vi "Get Installed Sections.vi"(8 "error in (no error)":errorcluster, 9 "Cached (F)":bool, 11 "Session in":refnum<k21>) -> (0 "error out":errorcluster, 2 "Software Components":T1[](array[typedef]) {"Visibility Type" items=["standard", "hidden", "system", "unknown", "startup", "image"]}, 3 "Session out":refnum<k21>)   [LabVIEW 2014, in "nisyscfg.lvlib"]
uses:
  nisyscfg.lvlib
  Software Extended.ctl
  Component Type.ctl
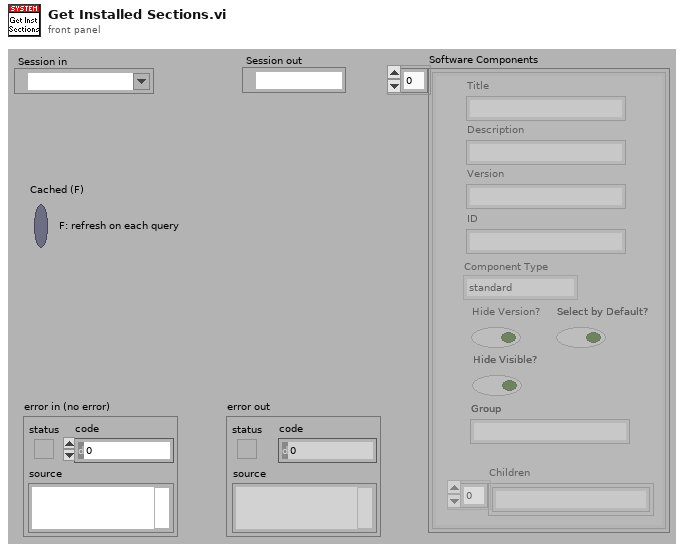
[diagram p1: front panel]
types:
  T1 = typedef "nisyscfg.lvlib/Software Extended.ctl" = cluster{"Description":string, "ID":string, "Version":string, "Title":string, "Visibility Type":T2, "Hide Version?":bool, "Children":string[], "Select by Default?":bool, "Hide Visible?":bool, "Group":string}
  T2 = typedef "nisyscfg.lvlib/Component Type.ctl" = u32
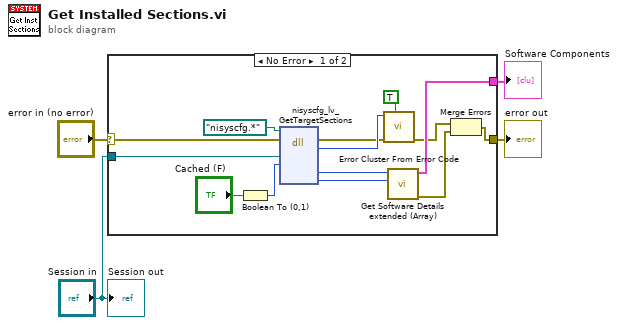
[diagram p0: block diagram]
diagram:
  n1 = case shown="No Error" "error in (no error)" {
    selector: "error in (no error)" -> [w15 w19]
    tunnel: [w9 _] -> w1
    tunnel: [w7 w19] -> w4
    tunnel: "Session in" -> [w14 _]
    frame No Error {
      n2 = Boolean To (0,1)(Boolean="Cached (F)") -> (0, 1=w16:i16)
      n3 = dll-call lib="nisyscfg.*" fn="nisyscfg_lv_GetTargetSections" label="GetTargetSections"(path in=path "nisyscfg.*", error in=w15, "system"=w14, "cached"=w16) -> (error out=w8:errorcluster, "result"=w18:i32, "sections"=w11:u64, "numSections"=w10:i32)  [unwired: 5 in, 1 out]
      n4 = call "Error Cluster From Error Code.vi"("show call chain? (False)"=TRUE, "error in (no error)"=w8, "error code (0)"=w18) -> ("error out"=w6:errorcluster)  [unwired: 6 in]
      n5 = call "Get Software Details extended (Array).vi"("Number of Elements"=w10, "Enumerator in"=w11) -> ("error out"=w5:errorcluster, "Software Components"=w9:T1[])  [unwired: 8 in]
      n6 = Merge Errors(w6, w5) -> (w7:errorcluster)
    }
    frame Error {
    }
  }
  "error out" <- w4
  "Software Components" <- w1
  "Session out" <- "Session in"
